vi "GetShaftSpeed.vi"(4 "Scan Period":dbl format="%.2f", 5 "Previous Scan Value":dbl format="%.2f", 6 "Present scan array":dbl[](array[numeric]) format="%.2f", 7 "Value to Output":dbl format="%.2f", 8 "Ch Description":T1={"Ch Name"="", "Type"="", "Function"=enum."Analogue Input", "Ch State"=enum."On", "Calibration type"="", "A"=0.0, "B"=0.0, "C"=0.0, "D"=0.0, "Comments"="", "Address"={"Main"=0, "Ch."=0, "Sub"=0, "Port Name"=""}, "String"="", "Duty"=65535} {"Duty" format="%016b"; "D" format="%#_5g"; "C" format="%#_5g"; "B" format="%#_5g"; "A" format="%#_5g"}, 9 "Ch names":string[](array[string])) -> (0 "Scan comment":string, 1 "Output":dbl format="%.3f", 3 "HelpText":string="Add helpful help text here!")   [LabVIEW 2022 SP3]
uses:
  ADAM Client/Sub VIs/ADAM Controls/Ch_description_ADAM.ctl
  ADAM Client/Sub VIs/ADAM Controls/Module_type_ADAM.ctl
  ADAM Client/Sub VIs/ADAM Controls/Function_ADAM.ctl
  ADAM Client/Sub VIs/ADAM Controls/Channel_State.ctl
  ADAM Client/Sub VIs/ADAM Controls/Calib_type_ADAM.ctl
  ADAM Client/Sub VIs/ADAM Controls/Address.ctl
panel:
  out "Read buffer":string
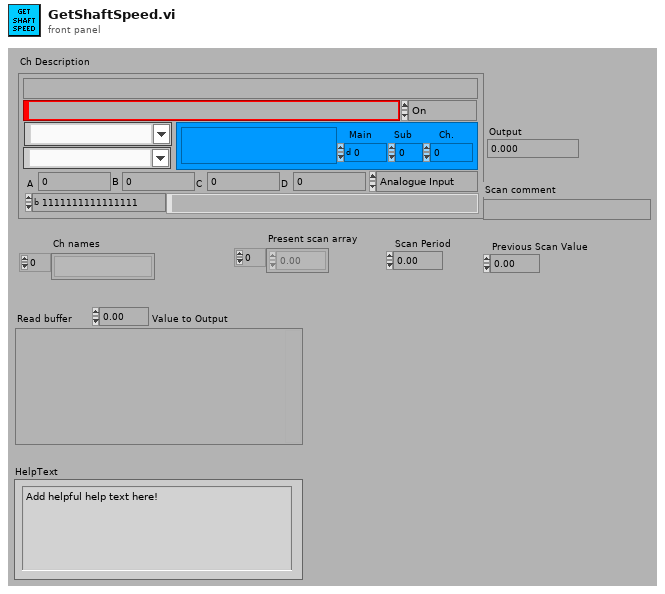
[diagram p1: front panel]
types:
  T1 = typedef "Ch_description_ADAM.ctl" = cluster{"Ch Name":string, "Type":T2, "Function":T3, "Ch State":T4, "Calibration type":T5, "A":dbl, "B":dbl, "C":dbl, "D":dbl, "Comments":string, "Address":T6, "String":string, "Duty":u16}
  T2 = typedef "Module_type_ADAM.ctl" = string
  T3 = typedef "Function_ADAM.ctl" = enum16{"Analogue Input", "Digital Input", "Event counter", "Event rate", "Analogue Output", "Digital Output", "Relay Output"}
  T4 = typedef "Channel_State.ctl" = enum16{"On", "Off", "Always On", "Always Off"}
  T5 = typedef "Calib_type_ADAM.ctl" = string
  T6 = typedef "Address.ctl" = cluster{"Main":i32, "Ch.":i32, "Sub":i32, "Port Name":string}
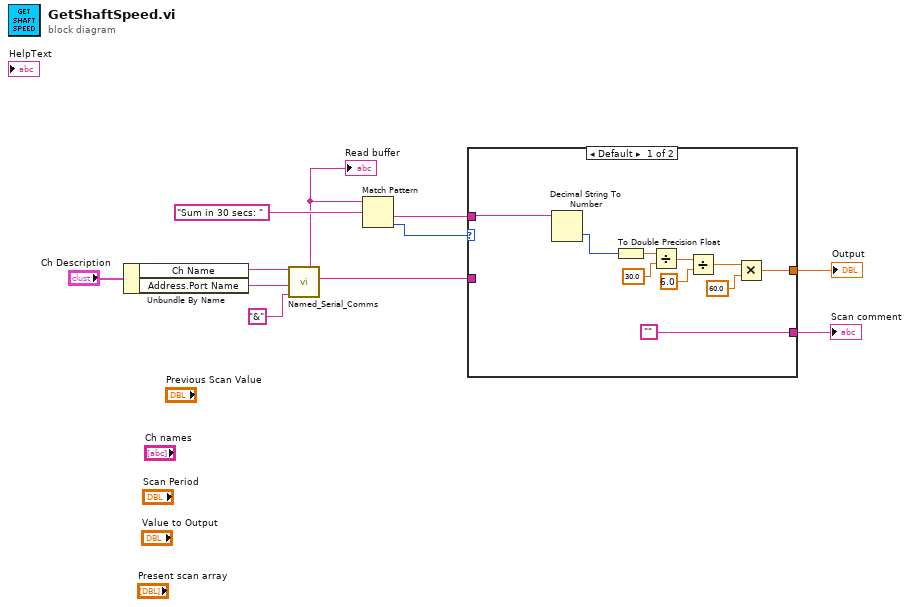
[diagram p0: block diagram]
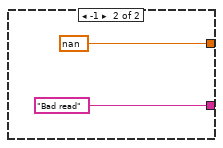
[diagram p2: hidden frame]
diagram:
  n1 = Unbundle By Name("Ch Description") -> ("Ch Name"=w1:string, "Address.Port Name"=w2:string)
  n2 = call "Named_Serial_Comms.vi"("Channel Name"=w1, "Port Name"=w2, "Term Grep"="&") -> ("Read"=w6:string)  [unwired: 6 in, 6 out]
  "Read buffer" <- w6
  n3 = Match Pattern(string=w6, regular expression="Sum in 30 secs: ") -> (after substring=w7:string, offset past match=w5:i32)  [unwired: 1 in, 2 out]
  n4 = case shown="Default" w5 {
    tunnel: ["" "Bad read" ("Read")] -> w9
    tunnel: w7 -> [w20 _]
    tunnel: w6 -> [_ _]
    tunnel: [w13 nan] -> w4
    frame Default {
      n5 = Decimal String To Number(string=w20) -> (number=w19:i32)  [unwired: 2 in, 1 out]
      n6 = To Double Precision Float(number=w19) -> (double precision float=w17:dbl)
      n7 = Divide(x=w17, y=30.0) -> (x/y=w15:dbl)
      n8 = Divide(x=w15, y=6.0) -> (x/y=w12:dbl)
      n9 = Multiply(x=w12, y=60.0) -> (x*y=w13:dbl)
    }
    frame -1 {
    }
  }
  "Output" <- w4
  "Scan comment" <- w9
